vi "H5Fis_hdf5.vi"(6 "error in (no error)":errorcluster, 9 "path":path) -> (0 "error out":errorcluster, 3 "Is HDF5":bool)   [LabVIEW 2017]
doc: "Determines whether a file is in the HDF5 format."
uses:
  <vilib>/UPVI/lvhdf5/hdf5.dll
panel:
  # "LVHDF5 Toolkit\nCopyright (c) 2005-2013 by Jason D. Sommerville\nCopyright (c) 2014 by UPVI, LLC.\n\nThis use and distribution of this file is governed by the terms found in \nLICENSE.txt distributed with this toolkit and installed at\n <user.lib>\\_lvhdf5\\LICENSE.txt"
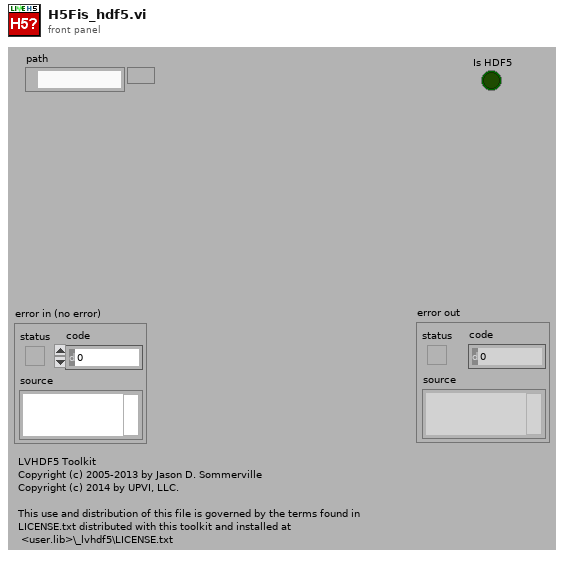
[diagram p1: front panel]
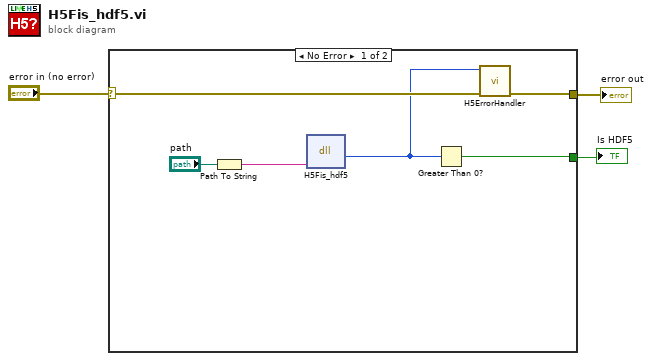
[diagram p0: block diagram]
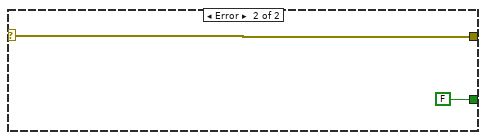
[diagram p2: hidden frame]
diagram:
  n1 = case shown="No Error" "error in (no error)" {
    selector: "error in (no error)" -> [w9 w11]
    tunnel: [w8 w11] -> w2
    tunnel: [w4 FALSE] -> w1
    frame No Error {
      n2 = Path To String(path="path") -> (string=w7:string)
      n3 = dll-call lib="C:/Program Files/National Instruments/LabVIEW 2017/vi.lib/UPVI/lvhdf5/hdf5.dll" fn="H5Fis_hdf5"("path"=w7) -> (w5:i32)  [unwired: 4 in, 2 out]
      n4 = Greater Than 0?(x=w5) -> (x > 0?=w4:bool)
      n5 = call <vilib>:"H5ErrorHandler.vi"("error in (no error)"=w9, "herr_t"=w5) -> ("error out"=w8:errorcluster)  [unwired: 3 in, 4 out]
    }
    frame Error {
    }
  }
  "error out" <- w2
  "Is HDF5" <- w1
